vi "TDMS_File_Setup.vi"(6 "Sensor IDs":variant[](array[variant]), 8 "error in (no error)":errorcluster, 9 "TestID":variant[](array[variant]), 10 "operation (0:open)":T1(ring), 11 "file path":path) -> (1 "error out":errorcluster, 2 "tdms file out":refnum<k34>)   [LabVIEW 2021]
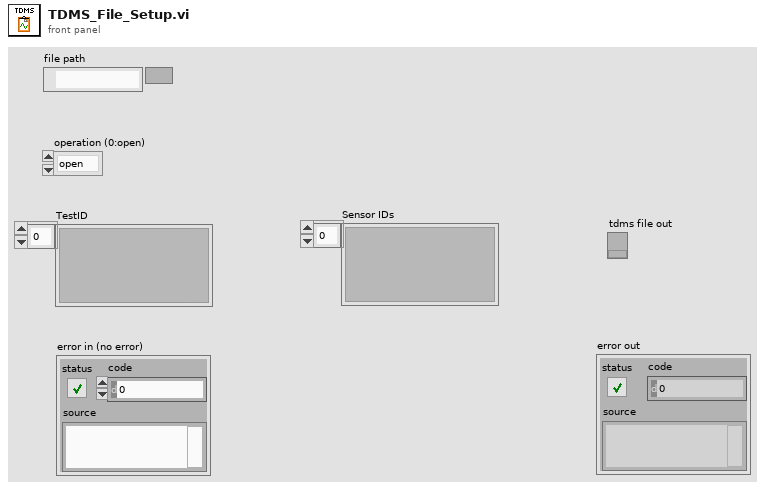
[diagram p1: front panel]
types:
  T1 = enum16{"open", "open or create", "create or replace", "create", "open (read-only)"}
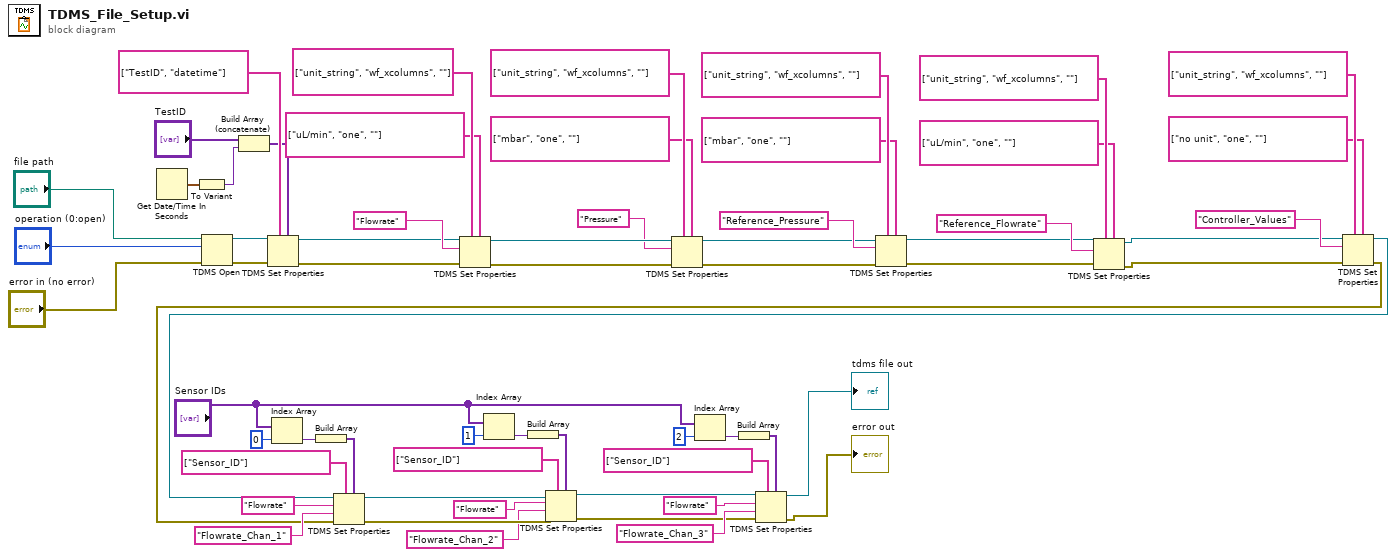
[diagram p0: block diagram]
diagram:
  n1 = Get Date/Time In Seconds() -> (seconds since 1Jan1904=w42:timestamp)
  n2 = To Variant(anything=w42) -> (Variant=w41:variant)
  n3 = TDMS Open(8:"error in (no error)", 10:"operation (0:open)", 11:"file path") -> (0:w59:errorcluster, 3:w58:refnum<k34>)  [unwired: 4 in]
  n4 = Build Array (concatenate)("TestID", w41) -> (w40:variant[])
  n5 = TDMS Set Properties(5:w40, 7:string[] ["TestID", "datetime"] ("property names"), 8:w59, 11:w58) -> (0:w56:errorcluster, 3:w54:refnum<k34>)  [unwired: 2 in, 2 out]
  n6 = Index Array(array="Sensor IDs", index=0) -> (element=w25:variant)
  n7 = Build Array(w25) -> (w24:variant[])
  n8 = TDMS Set Properties(5:string[] ["uL/min", "one", ""] ("property names"), 7:string[] ["unit_string", "wf_xcolumns", ""] ("property names"), 8:w56, 10:"Flowrate" ("group name"), 11:w54) -> (0:w55:errorcluster, 3:w53:refnum<k34>)  [unwired: 1 in, 2 out]
  n9 = Index Array(array="Sensor IDs", index=1) -> (element=w22:variant)
  n10 = Build Array(w22) -> (w17:variant[])
  n11 = TDMS Set Properties(5:string[] ["mbar", "one", ""] ("property names"), 7:string[] ["unit_string", "wf_xcolumns", ""] ("property names"), 8:w55, 10:"Pressure" ("group name"), 11:w53) -> (0:w6:errorcluster, 3:w5:refnum<k34>)  [unwired: 1 in, 2 out]
  n12 = Index Array(array="Sensor IDs", index=2) -> (element=w20:variant)
  n13 = Build Array(w20) -> (w18:variant[])
  n14 = TDMS Set Properties(5:string[] ["mbar", "one", ""] ("property names"), 7:string[] ["unit_string", "wf_xcolumns", ""] ("property names"), 8:w6, 10:"Reference_Pressure" ("group name"), 11:w5) -> (0:w3:errorcluster, 3:w4:refnum<k34>)  [unwired: 1 in, 2 out]
  n15 = TDMS Set Properties(5:string[] ["uL/min", "one", ""] ("property names"), 7:string[] ["unit_string", "wf_xcolumns", ""] ("property names"), 8:w3, 10:"Reference_Flowrate" ("group name"), 11:w4) -> (0:w2:errorcluster, 3:w1:refnum<k34>)  [unwired: 1 in, 2 out]
  n16 = TDMS Set Properties(5:string[] ["no unit", "one", ""] ("property names"), 7:string[] ["unit_string", "wf_xcolumns", ""] ("property names"), 8:w2, 10:"Controller_Values" ("group name"), 11:w1) -> (0:w14:errorcluster, 3:w13:refnum<k34>)  [unwired: 1 in, 2 out]
  n17 = TDMS Set Properties(5:w24, 7:string[] ["Sensor_ID"] ("property names"), 8:w14, 9:"Flowrate_Chan_1" ("channel name"), 10:"Flowrate" ("group name"), 11:w13) -> (0:w32:errorcluster, 3:w30:refnum<k34>)  [unwired: 2 out]
  n18 = TDMS Set Properties(5:w17, 7:string[] ["Sensor_ID"] ("property names"), 8:w32, 9:"Flowrate_Chan_2" ("channel name"), 10:"Flowrate" ("group name"), 11:w30) -> (0:w31:errorcluster, 3:w29:refnum<k34>)  [unwired: 2 out]
  n19 = TDMS Set Properties(5:w18, 7:string[] ["Sensor_ID"] ("property names"), 8:w31, 9:"Flowrate_Chan_3" ("channel name"), 10:"Flowrate" ("group name"), 11:w29) -> (0:→"error out":errorcluster, 3:→"tdms file out":refnum<k34>)  [unwired: 2 out]
